vi "arduino_data_and_filters_V2_subVI.vi"(7 "loop iteration number":i32, 8 "arduino 1-6 address and errors":T3, 11 "arduinos on?":bool) -> (0 "arduino 1-6 addresses and errors out":T2, 1 "arduino 1-6 data out":T1, 3 "arduinos on? output":bool)   [LabVIEW 2014]
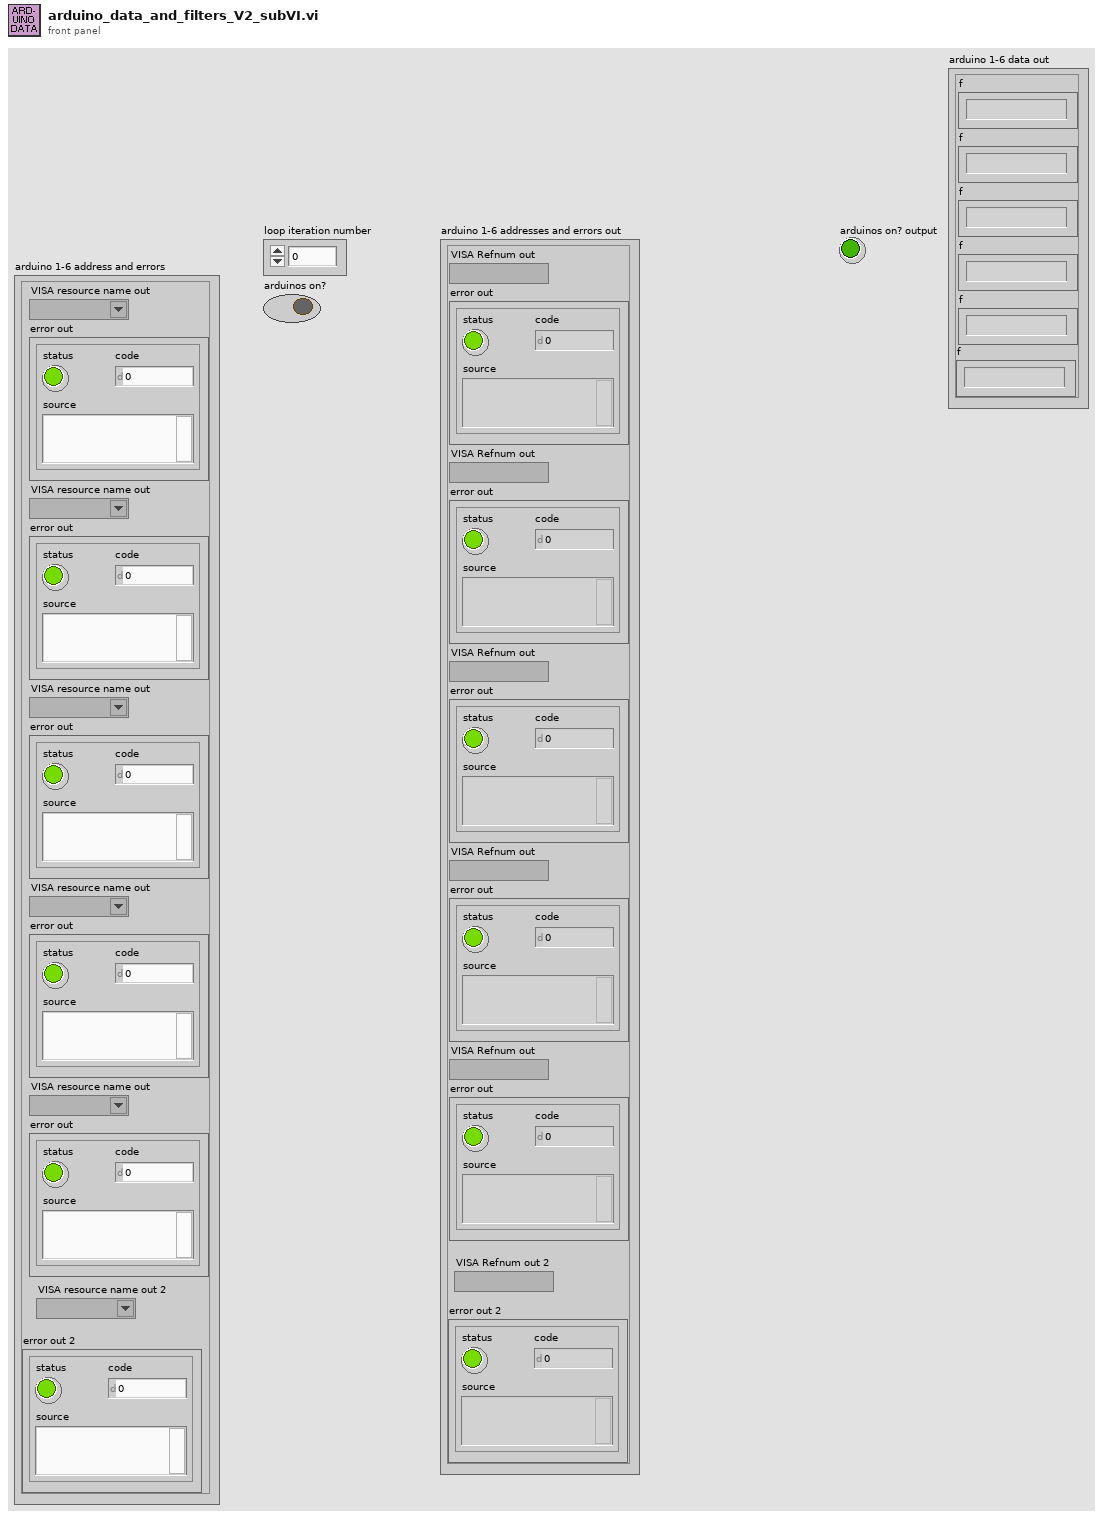
[diagram p1: front panel]
types:
  T1 = cluster{"f":string, "f":string, "f":string, "f":string, "f":string, "f":string}
  T2 = cluster{"VISA Refnum out":refnum<visa-resource-name>, "error out":errorcluster, "VISA Refnum out":refnum<visa-resource-name>, "error out":errorcluster, "VISA Refnum out":refnum<visa-resource-name>, "error out":errorcluster, "VISA Refnum out":refnum<visa-resource-name>, "error out":errorcluster, "VISA Refnum out":refnum<visa-resource-name>, "error out":errorcluster, "VISA Refnum out 2":refnum<visa-resource-name>, "error out 2":errorcluster}
  T3 = cluster{"VISA resource name out":refnum<visa-resource-name>, "error out":errorcluster, "VISA resource name out":refnum<visa-resource-name>, "error out":errorcluster, "VISA resource name out":refnum<visa-resource-name>, "error out":errorcluster, "VISA resource name out":refnum<visa-resource-name>, "error out":errorcluster, "VISA resource name out":refnum<visa-resource-name>, "error out":errorcluster, "VISA resource name out 2":refnum<visa-resource-name>, "error out 2":errorcluster}
  T4 = cluster{"f":string, "f":string, "f":string, "f":string, "f":string, "f 2":string}
  T5 = cluster{"VISA Refnum out":refnum<visa-resource-name>, "error out":errorcluster, "VISA Refnum out":refnum<visa-resource-name>, "error out":errorcluster, "VISA Refnum out":refnum<visa-resource-name>, "error out":errorcluster, "VISA Refnum out":refnum<visa-resource-name>, "error out":errorcluster, "VISA Refnum out":refnum<visa-resource-name>, "error out":errorcluster, "VISA Refnum out":refnum<visa-resource-name>, "error out":errorcluster}
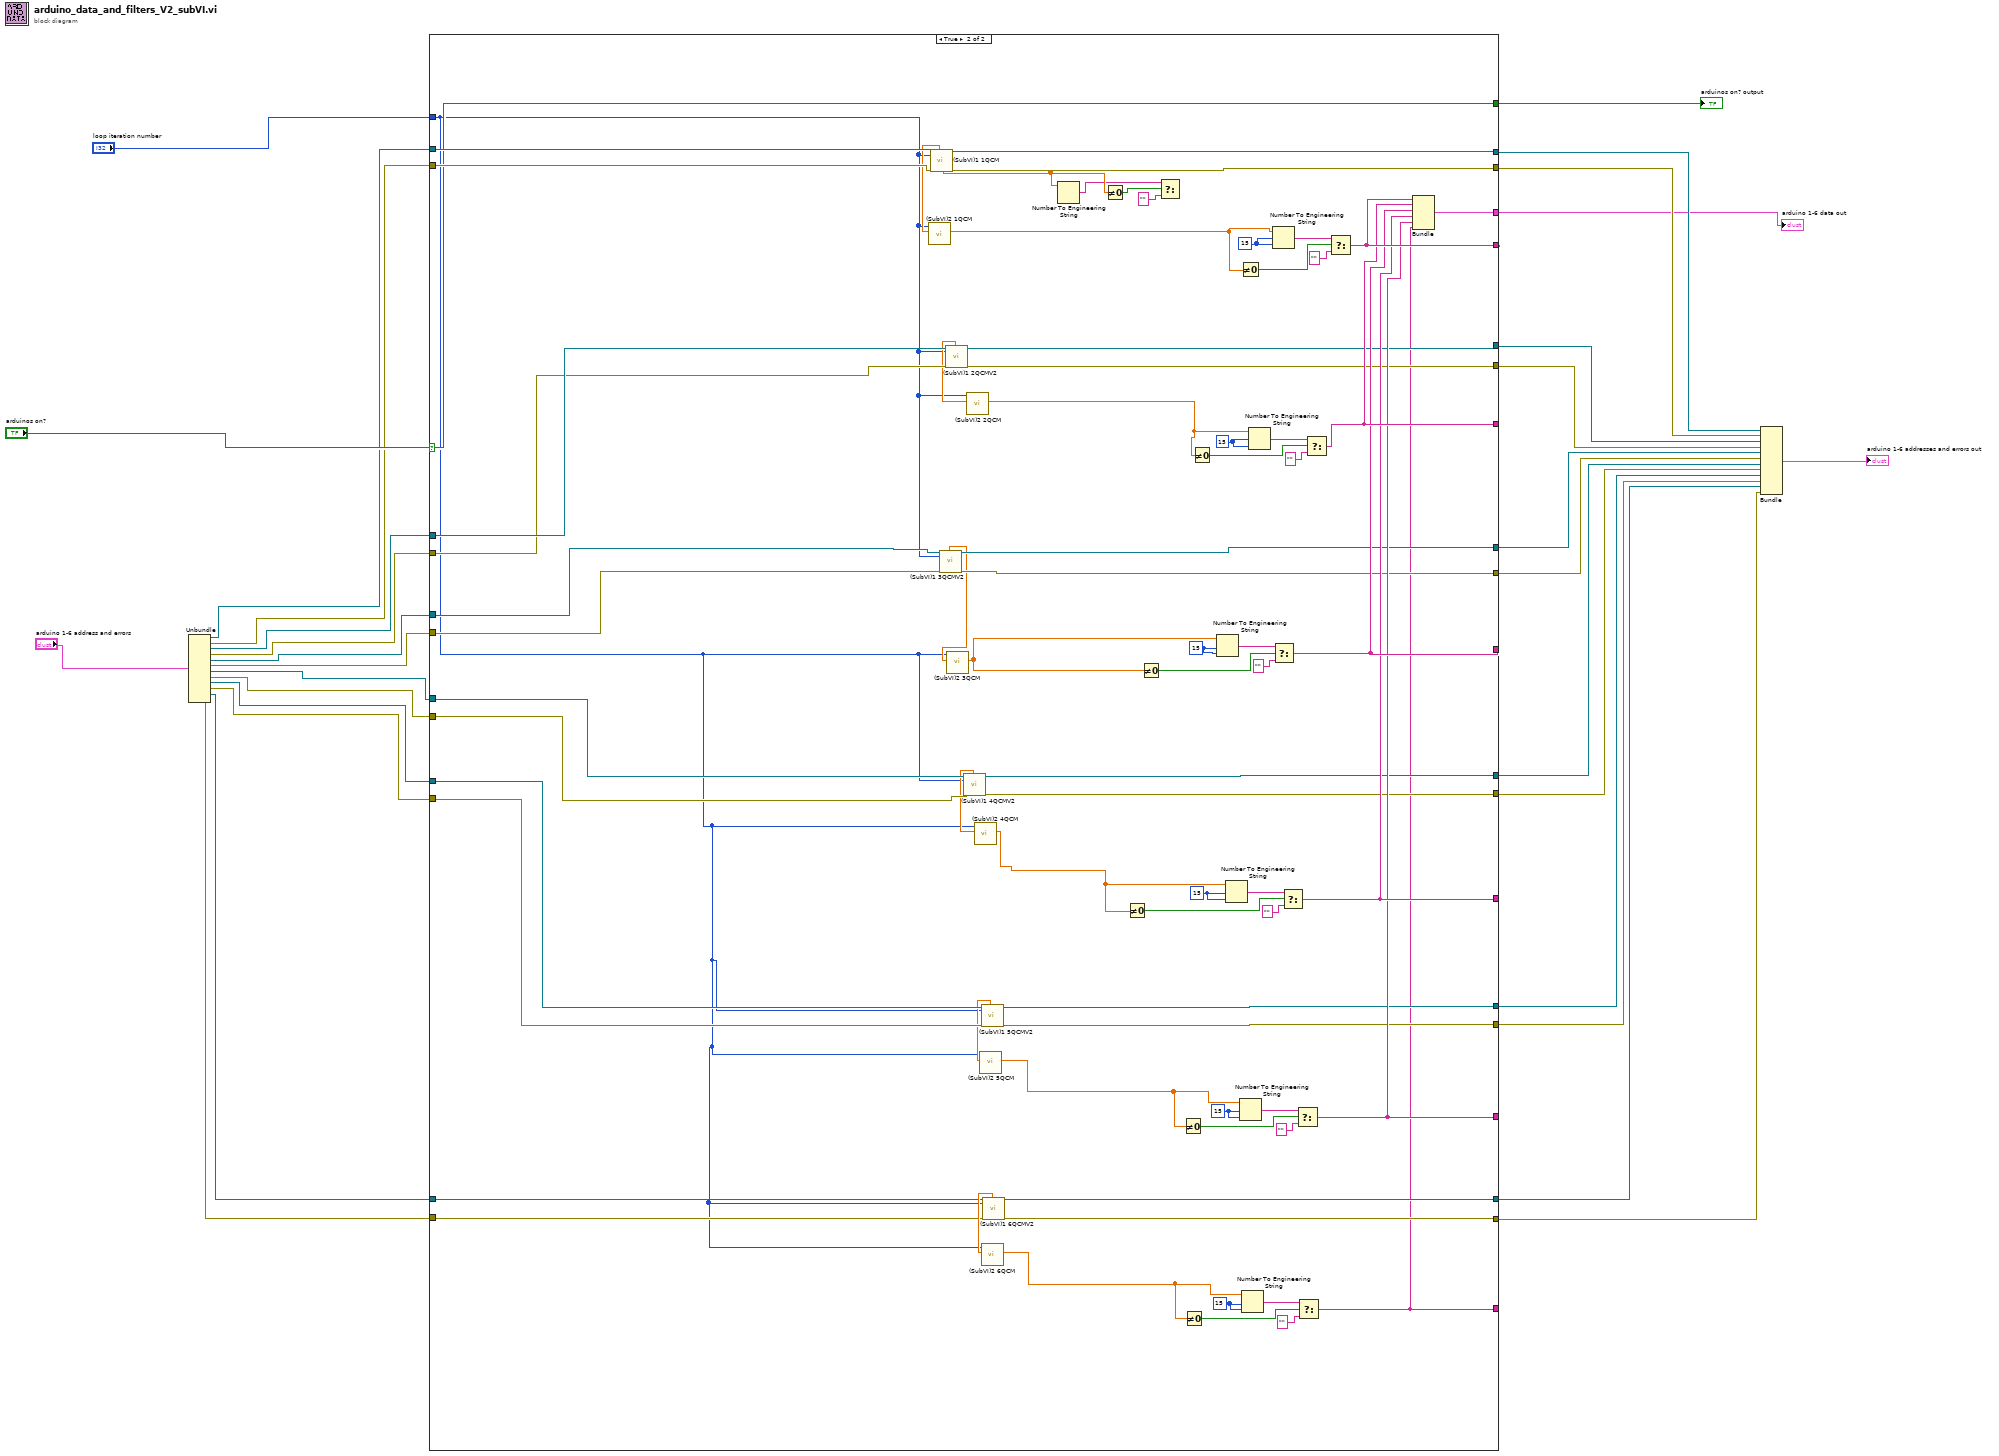
[diagram p0: block diagram]
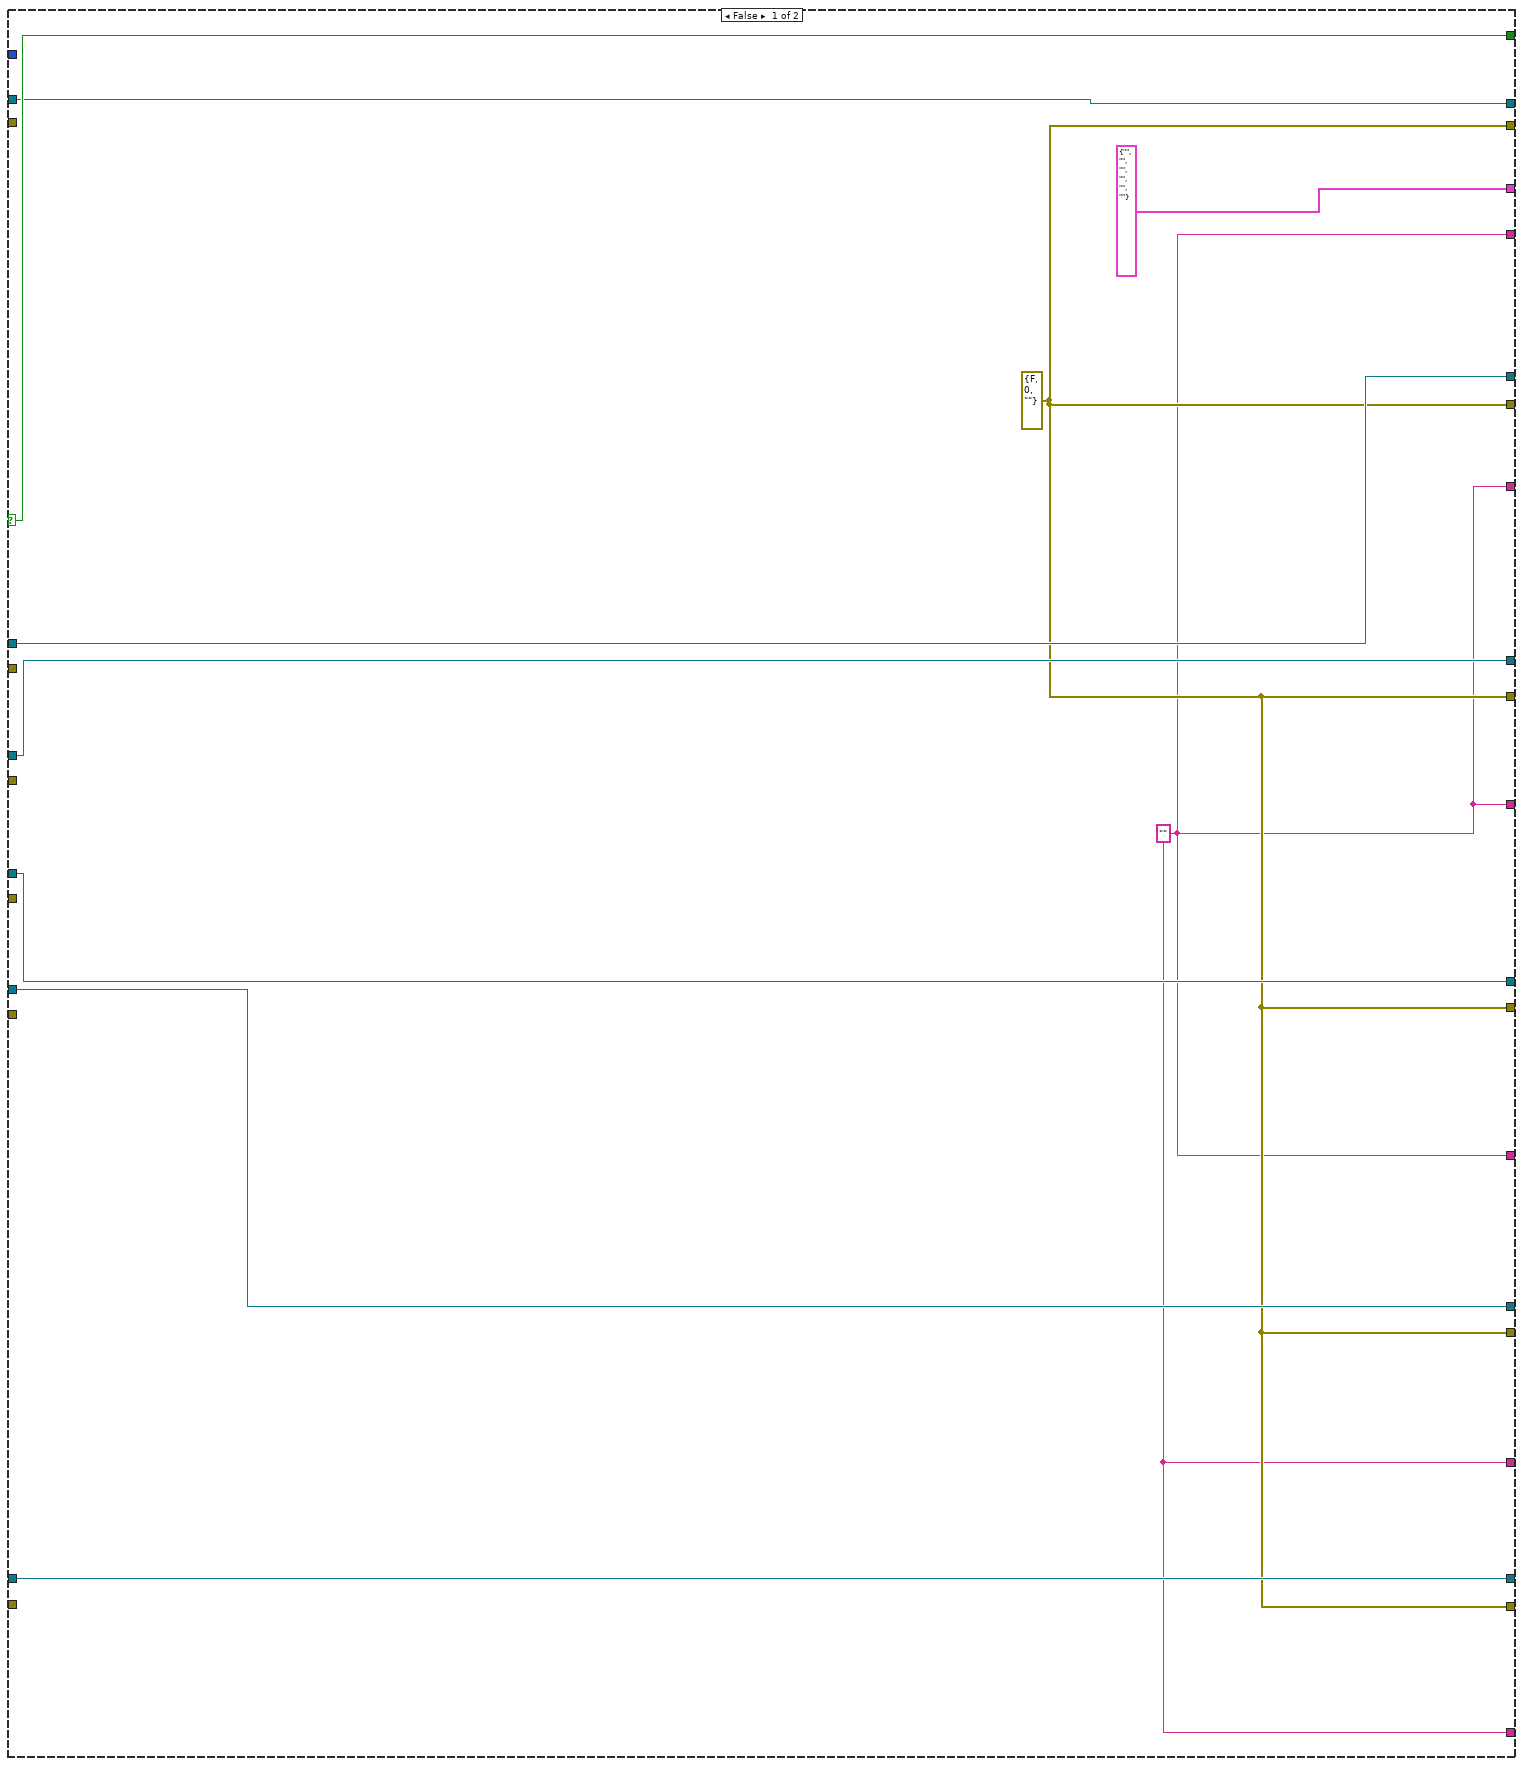
[diagram p2: hidden frame]
diagram:
  n1 = Unbundle("arduino 1-6 address and errors") -> ("VISA resource name out"=w14:refnum<visa-resource-name>, "error out"=w13:errorcluster, "VISA resource name out"=w12:refnum<visa-resource-name>, "error out"=w11:errorcluster, "VISA resource name out"=w10:refnum<visa-resource-name>, "error out"=w9:errorcluster, "VISA resource name out"=w8:refnum<visa-resource-name>, "error out"=w7:errorcluster, "VISA resource name out"=w6:refnum<visa-resource-name>, "error out"=w5:errorcluster, "VISA resource name out 2"=w4:refnum<visa-resource-name>, "error out 2"=w3:errorcluster)
  n2 = case shown="True" "arduinos on?" {
    selector: "arduinos on?" -> [w40 w109]
    tunnel: [w40 w109] -> w17
    tunnel: w14 -> [w39 w112]
    tunnel: w13 -> [_ w113]
    tunnel: [w32 w111] -> w27
    tunnel: [w39 w110] -> w28
    tunnel: "loop iteration number" -> [_ w41]
    tunnel: w12 -> [w38 w83]
    tunnel: w11 -> [_ w82]
    tunnel: [w38 w77] -> w26
    tunnel: [w32 w76] -> w25
    tunnel: w10 -> [w37 w74]
    tunnel: w9 -> [_ w72]
    tunnel: [w37 w73] -> w24
    tunnel: [w32 w71] -> w23
    tunnel: w8 -> [w36 w66]
    tunnel: w7 -> [_ w68]
    tunnel: w6 -> [w35 w63]
    tunnel: w5 -> [_ w60]
    tunnel: [w32 w67] -> w21
    tunnel: [w36 w69] -> w22
    tunnel: [w35 w62] -> w20
    tunnel: [w32 w61] -> w19
    tunnel: [w31 w89] -> _
    tunnel: [w31 w88] -> _
    tunnel: [w31 w87] -> _
    tunnel: [w31 w85] -> _
    tunnel: [w31 w86] -> _
    tunnel: [T4 {"f"="", "f"="", "f"="", "f"="", "f"="", "f 2"=""} w84] -> w16
    tunnel: w4 -> [w33 w46]
    tunnel: w3 -> [_ w45]
    tunnel: [w33 w44] -> w1
    tunnel: [w32 w43] -> w2
    tunnel: [w31 w42] -> _
    frame False {
      w31 = "" ("f")
      w32 = errorcluster {"status"=FALSE, "code"=0, "source"=""} ("error out")
    }
    frame True {
      w52 = i16 15 ("width (-)")
      w53 = i16 15 ("width (-)")
      w54 = i16 15 ("width (-)")
      w55 = i16 15 ("width (-)")
      w56 = i16 15 ("width (-)")
      w57 = i16 15 ("width (-)")
      n3 = call "(SubVI)1 1QCM.vi"("VISA Refnum in"=w112, "main loop iteration number"=w41, "error in (no error)"=w113) -> ("Freq out"=w80:dbl, "unfiltered freq out"=w108:dbl, "VISA Refnum out"=w110:refnum<visa-resource-name>, "error out"=w111:errorcluster)  [unwired: 11 in, 2 out]
      n4 = call "(SubVI)2 1QCM.vi"("Numeric in"=w80, "Numeric"=w41) -> ("Mean"=w81:dbl)  [unwired: 6 in, 3 out]
      n5 = call "(SubVI)1 3QCMV2.vi"("VISA Refnum in"=w74, "main loop iteration number"=w41, "error in (no error)"=w72) -> ("Freq out"=w70:dbl, "VISA Refnum out"=w73:refnum<visa-resource-name>, "error out"=w71:errorcluster)  [unwired: 11 in, 3 out]
      n6 = call "(SubVI)1 2QCMV2.vi"("VISA Refnum in"=w83, "main loop iteration number"=w41, "error in (no error)"=w82) -> ("Freq out"=w79:dbl, "VISA Refnum out"=w77:refnum<visa-resource-name>, "error out"=w76:errorcluster)  [unwired: 11 in, 3 out]
      n7 = call "(SubVI)2 3QCM.vi"("Numeric in"=w70, "Numeric"=w41) -> ("Mean"=w75:dbl)  [unwired: 6 in, 3 out]
      n8 = call "(SubVI)1 4QCMV2.vi"("VISA Refnum in"=w66, "main loop iteration number"=w41, "error in (no error)"=w68) -> ("Freq out"=w64:dbl, "VISA Refnum out"=w69:refnum<visa-resource-name>, "error out"=w67:errorcluster)  [unwired: 11 in, 3 out]
      n9 = call "(SubVI)2 2QCM.vi"("Numeric in"=w79, "Numeric"=w41) -> ("Mean"=w78:dbl)  [unwired: 6 in, 3 out]
      n10 = call "(SubVI)2 4QCM.vi"("Numeric in"=w64, "Numeric"=w41) -> ("Mean"=w65:dbl)  [unwired: 6 in, 3 out]
      n11 = call "(SubVI)1 5QCMV2.vi"("VISA Refnum in"=w63, "main loop iteration number"=w41, "error in (no error)"=w60) -> ("Freq out"=w59:dbl, "VISA Refnum out"=w62:refnum<visa-resource-name>, "error out"=w61:errorcluster)  [unwired: 11 in, 3 out]
      n12 = call "(SubVI)2 5QCM.vi"("Numeric in"=w59, "Numeric"=w41) -> ("Mean"=w58:dbl)  [unwired: 6 in, 3 out]
      n13 = call "(SubVI)1 6QCMV2.vi"("VISA Refnum in"=w46, "main loop iteration number"=w41, "error in (no error)"=w45) -> ("Freq out"=w50:dbl, "VISA Refnum out"=w44:refnum<visa-resource-name>, "error out"=w43:errorcluster)  [unwired: 11 in, 3 out]
      n14 = call "(SubVI)2 6QCM.vi"("Numeric in"=w50, "Numeric"=w41) -> ("Mean"=w51:dbl)  [unwired: 6 in, 3 out]
      n15 = Number To Engineering String(4:w108) -> (0:w106:string)  [unwired: 3 in]
      n16 = Not Equal To 0?(x=w108) -> (x != 0?=w107:bool)
      n17 = Not Equal To 0?(x=w65) -> (x != 0?=w93:bool)
      n18 = Not Equal To 0?(x=w75) -> (x != 0?=w98:bool)
      n19 = Select(t=w106, s=w107, f="") -> ()  [unwired: 1 out]
      n20 = Not Equal To 0?(x=w58) -> (x != 0?=w92:bool)
      n21 = Not Equal To 0?(x=w51) -> (x != 0?=w47:bool)
      n22 = Not Equal To 0?(x=w78) -> (x != 0?=w99:bool)
      n23 = Number To Engineering String(2:w55, 3:w55, 4:w75) -> (0:w97:string)  [unwired: 1 in]
      n24 = Number To Engineering String(2:w54, 3:w54, 4:w65) -> (0:w94:string)  [unwired: 1 in]
      n25 = Not Equal To 0?(x=w81) -> (x != 0?=w102:bool)
      n26 = Number To Engineering String(2:w53, 3:w53, 4:w58) -> (0:w91:string)  [unwired: 1 in]
      n27 = Number To Engineering String(2:w52, 3:w52, 4:w51) -> (0:w48:string)  [unwired: 1 in]
      n28 = Number To Engineering String(2:w56, 3:w56, 4:w78) -> (0:w100:string)  [unwired: 1 in]
      n29 = Number To Engineering String(2:w57, 3:w57, 4:w81) -> (0:w103:string)  [unwired: 1 in]
      n30 = Select(t=w97, s=w98, f="") -> (s? t:f=w87:string)
      n31 = Select(t=w94, s=w93, f="") -> (s? t:f=w86:string)
      n32 = Select(t=w91, s=w92, f="") -> (s? t:f=w85:string)
      n33 = Select(t=w48, s=w47, f="") -> (s? t:f=w42:string)
      n34 = Select(t=w100, s=w99, f="") -> (s? t:f=w88:string)
      n35 = Select(t=w103, s=w102, f="") -> (s? t:f=w89:string)
      n36 = Bundle("f"=w89, "f"=w88, "f"=w87, "f"=w86, "f"=w85, "f"=w42) -> (w84:T1)  [unwired: 1 in]
    }
  }
  "arduinos on? output" <- w17
  "arduino 1-6 data out" <- w16
  n37 = Bundle("VISA Refnum out"=w28, "error out"=w27, "VISA Refnum out"=w26, "error out"=w25, "VISA Refnum out"=w24, "error out"=w23, "VISA Refnum out"=w22, "error out"=w21, "VISA Refnum out"=w20, "error out"=w19, "VISA Refnum out"=w1, "error out"=w2) -> (→"arduino 1-6 addresses and errors out":T5)  [unwired: 1 in]
